vi "extract deleted folders.vi"(1 "Input Array":path[](array[path])) -> (0 "Deleted Folders":path[](array[path]))   [LabVIEW 2011]
doc: "This VI is necessary to remove the empty folders from the input array so that only the deleted folders are listed in the output array."
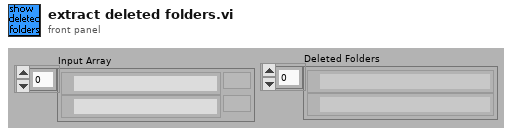
[diagram p1: front panel]
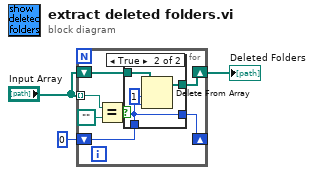
[diagram p0: block diagram]
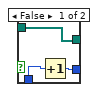
[diagram p2: hidden frame]
diagram:
  n1 = for {
    tunnel: "Input Array" -> [w9] mode=indexing
    shift-right: [w7] -> w3
    shift-left: "Input Array" -> [w6]
    shift-right: [w4] -> _
    shift-left: 0 -> [w5]
    n2 = Equal?(x=w9, y=path "") -> (x = y?=w10:bool)
    n3 = case shown="True" w10 {
      tunnel: [w13 w16] -> w7
      tunnel: w6 -> [w13 w15]
      tunnel: w5 -> [w11 w14]
      tunnel: [w12 w14] -> w4
      frame False {
        n4 = Increment(x=w11) -> (x+1=w12:i32)
      }
      frame True {
        n5 = Delete From Array(array=w15, length=1 ("Length"), index=w14) -> (array with subset deleted=w16:path[])  [unwired: 1 out]
      }
    }
  }
  "Deleted Folders" <- w3
